vi "Read from Hardware.vi"(8 "error in":errorcluster, 10 "Values in":dbl[](array[numeric]), 11 "Rx Execution Unit Implementation in":refnum<class "Rx Execution Unit.lvclass">) -> (0 "error out":errorcluster, 2 "Values out":dbl[](array[numeric]), 3 "Rx Execution Unit Implementation out":refnum<class "Rx Execution Unit.lvclass">)   [LabVIEW 2020, in "afdx_custom_device Engine.lvlib" / "Implementation.lvlib" / "Rx Execution Unit.lvclass"]
uses:
  Rx Execution Unit.lvclass
  AIM LabVIEW src/src/AIM664LV.lvlib
  afdx_custom_device Engine.lvlib
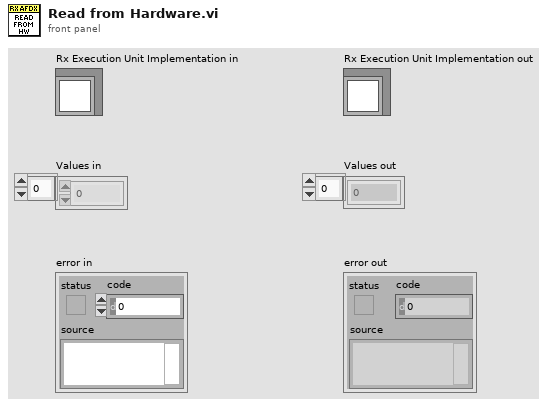
[diagram p1: front panel]
types:
  T1 = cluster{"TotalByteCount":u32[], "FrameGoodCount":u32[], "FrameErrorCount":u32[], "BytesPerSecond":u32[], "FramesPerSecond":u32[], "PhysErrorCount":u32[], "PreamErrorCount":u32[], "UnaligErrorCount":u32[], "CRCErrorCount":u32[], "IFGErrorCount":u32[], "IPErrorCount":u32[], "MACErrorCount":u32[], "NoSfdErrorCount":u32[], "VLLenErrorCount":u32[], "SNIntegrityErrorCount":u32[], "TrafShapingViolationCount":u32[], "MAC1Short":u32[], "MAC64To127Count":u32[], "MAC128To255Count":u32[], "MAC256To511Count":u32[], "MAC512To1023Count":u32[], "MAC1024To1518Count":u32[], "MACLong":u32[]}
  T2 = cluster{"MonStatus":u32, "FramesCaptured":u32, "BytesRecordedHiPart":u32, "BytesRecordedLoPart":u32}
  T3 = cluster{"EntryRead":u32, "BytesRead":u32, "Synchronized":u32, "ReadBuffer":u8[]}
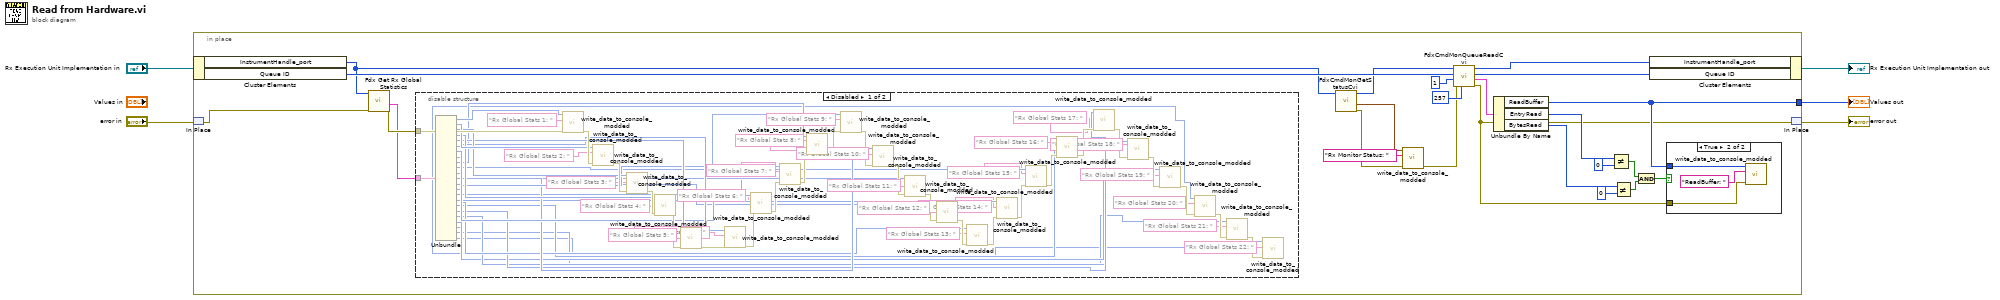
[diagram p0: block diagram]
diagram:
  n1 = in-place {
    in-place-border: [w19] -> w1
    n2 = in-place-cluster #1("Rx Execution Unit Implementation in") -> ("InstrumentHandle_port"=w7:u32, "Queue ID"=w29:u32)
    n3 = in-place-match #2("error in") -> (w14:errorcluster)
    n4 = call "Fdx Get Rx Global Statistics.vi"("error in"=w14, "InstrumentHandle_port in"=w7) -> ("error out"=w8:errorcluster, "GlobalStat Out"=w6:T1)  [unwired: 7 in, 1 out]
    n5 = disable-structure shown="Disabled" {
      disable-tunnel: w8 -> [w99 _]
      disable-tunnel: w6 -> [w97 _]
      frame Disabled {
        n6 = Unbundle(w97) -> ("TotalByteCount"=w96:u32[], "FrameGoodCount"=w89:u32[], "FrameErrorCount"=w88:u32[], "BytesPerSecond"=w87:u32[], "FramesPerSecond"=w86:u32[], "PhysErrorCount"=w85:u32[], "PreamErrorCount"=w84:u32[], "UnaligErrorCount"=w77:u32[], "CRCErrorCount"=w76:u32[], "IFGErrorCount"=w75:u32[], "IPErrorCount"=w74:u32[], "MACErrorCount"=w73:u32[], "NoSfdErrorCount"=w72:u32[], "VLLenErrorCount"=w65:u32[], "SNIntegrityErrorCount"=w64:u32[], "TrafShapingViolationCount"=w63:u32[], "MAC1Short"=w62:u32[], "MAC64To127Count"=w61:u32[], "MAC128To255Count"=w60:u32[], "MAC256To511Count"=w55:u32[], "MAC512To1023Count"=w54:u32[], "MAC1024To1518Count"=w53:u32[], "MACLong"=w52:u32[])
        n7 = call "write_data_to_console_modded.vi"("error in"=w99, "Tag"="Rx Global Stats 1: ", "Data"=w96) -> ("error out"=w95:errorcluster)  [unwired: 8 in]
        n8 = call "write_data_to_console_modded.vi"("error in"=w95, "Tag"="Rx Global Stats 2: ", "Data"=w89) -> ("error out"=w94:errorcluster)  [unwired: 8 in]
        n9 = call "write_data_to_console_modded.vi"("error in"=w94, "Tag"="Rx Global Stats 3: ", "Data"=w88) -> ("error out"=w93:errorcluster)  [unwired: 8 in]
        n10 = call "write_data_to_console_modded.vi"("error in"=w93, "Tag"="Rx Global Stats 4: ", "Data"=w87) -> ("error out"=w92:errorcluster)  [unwired: 8 in]
        n11 = call "write_data_to_console_modded.vi"("error in"=w92, "Tag"="Rx Global Stats 5: ", "Data"=w86) -> ("error out"=w91:errorcluster)  [unwired: 8 in]
        n12 = call "write_data_to_console_modded.vi"("error in"=w91, "Tag"="Rx Global Stats 5.5: ", "Data"=w85) -> ("error out"=w90:errorcluster)  [unwired: 8 in]
        n13 = call "write_data_to_console_modded.vi"("error in"=w90, "Tag"="Rx Global Stats 6: ", "Data"=w84) -> ("error out"=w83:errorcluster)  [unwired: 8 in]
        n14 = call "write_data_to_console_modded.vi"("error in"=w83, "Tag"="Rx Global Stats 7: ", "Data"=w77) -> ("error out"=w82:errorcluster)  [unwired: 8 in]
        n15 = call "write_data_to_console_modded.vi"("error in"=w82, "Tag"="Rx Global Stats 8: ", "Data"=w76) -> ("error out"=w81:errorcluster)  [unwired: 8 in]
        n16 = call "write_data_to_console_modded.vi"("error in"=w81, "Tag"="Rx Global Stats 9: ", "Data"=w75) -> ("error out"=w80:errorcluster)  [unwired: 8 in]
        n17 = call "write_data_to_console_modded.vi"("error in"=w80, "Tag"="Rx Global Stats 10: ", "Data"=w74) -> ("error out"=w79:errorcluster)  [unwired: 8 in]
        n18 = call "write_data_to_console_modded.vi"("error in"=w79, "Tag"="Rx Global Stats 11: ", "Data"=w73) -> ("error out"=w78:errorcluster)  [unwired: 8 in]
        n19 = call "write_data_to_console_modded.vi"("error in"=w78, "Tag"="Rx Global Stats 12: ", "Data"=w72) -> ("error out"=w71:errorcluster)  [unwired: 8 in]
        n20 = call "write_data_to_console_modded.vi"("error in"=w71, "Tag"="Rx Global Stats 13: ", "Data"=w65) -> ("error out"=w70:errorcluster)  [unwired: 8 in]
        n21 = call "write_data_to_console_modded.vi"("error in"=w70, "Tag"="Rx Global Stats 14: ", "Data"=w64) -> ("error out"=w69:errorcluster)  [unwired: 8 in]
        n22 = call "write_data_to_console_modded.vi"("error in"=w69, "Tag"="Rx Global Stats 15: ", "Data"=w63) -> ("error out"=w68:errorcluster)  [unwired: 8 in]
        n23 = call "write_data_to_console_modded.vi"("error in"=w68, "Tag"="Rx Global Stats 16: ", "Data"=w62) -> ("error out"=w67:errorcluster)  [unwired: 8 in]
        n24 = call "write_data_to_console_modded.vi"("error in"=w67, "Tag"="Rx Global Stats 17: ", "Data"=w61) -> ("error out"=w66:errorcluster)  [unwired: 8 in]
        n25 = call "write_data_to_console_modded.vi"("error in"=w66, "Tag"="Rx Global Stats 18: ", "Data"=w60) -> ("error out"=w59:errorcluster)  [unwired: 8 in]
        n26 = call "write_data_to_console_modded.vi"("error in"=w59, "Tag"="Rx Global Stats 19: ", "Data"=w55) -> ("error out"=w58:errorcluster)  [unwired: 8 in]
        n27 = call "write_data_to_console_modded.vi"("error in"=w58, "Tag"="Rx Global Stats 20: ", "Data"=w54) -> ("error out"=w57:errorcluster)  [unwired: 8 in]
        n28 = call "write_data_to_console_modded.vi"("error in"=w57, "Tag"="Rx Global Stats 21: ", "Data"=w53) -> ("error out"=w56:errorcluster)  [unwired: 8 in]
        n29 = call "write_data_to_console_modded.vi"("error in"=w56, "Tag"="Rx Global Stats 22: ", "Data"=w52) -> ()  [unwired: 8 in, 1 out]
      }
      frame Enabled {
      }
    }
    n30 = call "FdxCmdMonGetStatusCvi.vi"("InstrumentHandle_port in"=w7) -> ("error out"=w12:errorcluster, "MonStatus"=w10:T2, "InstrumentHandle_port out"=w13:u32)  [unwired: 8 in]
    n31 = call "write_data_to_console_modded.vi"("error in"=w12, "Tag"="Rx Monitor Status: ", "Data"=w10) -> ("error out"=w11:errorcluster)  [unwired: 8 in]
    n32 = call "FdxCmdMonQueueReadCvi.vi"("MaxReadBytes"=u32 257, "error in"=w11, "EntryCount"=u32 1 ("EntryCount (1)"), "QueueId"=w29, "InstrumentHandle_port"=w13) -> ("error out"=w16:errorcluster, "QueueReadOut"=w25:T3, "QueueIdOut"=w28:u32, "InstrumentHandle_port"=w27:u32)  [unwired: 3 in]
    n33 = Unbundle By Name(w25) -> ("ReadBuffer"=w19:u8[], "EntryRead"=w17:u32, "BytesRead"=w18:u32)
    n34 = Not Equal?(x=w17, y=u32 0) -> (x != y?=w24:bool)
    n35 = Not Equal?(x=w18, y=u32 0) -> (x != y?=w23:bool)
    n36 = And(x=w24, y=w23) -> (x .and. y?=w20:bool)
    n37 = in-place-cluster #1("InstrumentHandle_port"=w27, "Queue ID"=w28) -> (→"Rx Execution Unit Implementation out":refnum<class "Rx Execution Unit.lvclass">)
    n38 = case shown="True" w20 {
      tunnel: w19 -> [_ w102]
      tunnel: w16 -> [_ w100]
      frame False {
      }
      frame True {
        n39 = call "write_data_to_console_modded.vi"("error in"=w100, "Tag"="ReadBuffer: ", "Data"=w102) -> ()  [unwired: 8 in, 1 out]
      }
    }
    n40 = in-place-match #2(w16) -> (→"error out":errorcluster)
  }
  "Values out" <- w1
